vi "Read Array Of Tag Elements.vi"(6 "error text in":string, 8 "error in":errorcluster, 10 "tag name":string, 11 "node in":refnum<k20>) -> (0 "error out":errorcluster, 3 "array of elements":refnum<k20>[](array[refnum]))   [LabVIEW 2020, in "AIM ARINC 664 Import.lvlib"]
uses:
  AIM ARINC 664 Import.lvlib
  <resource>/objmgr/DOMUserDefRef.rc
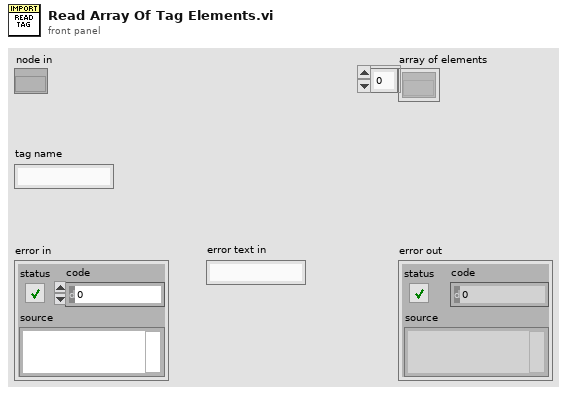
[diagram p1: front panel]
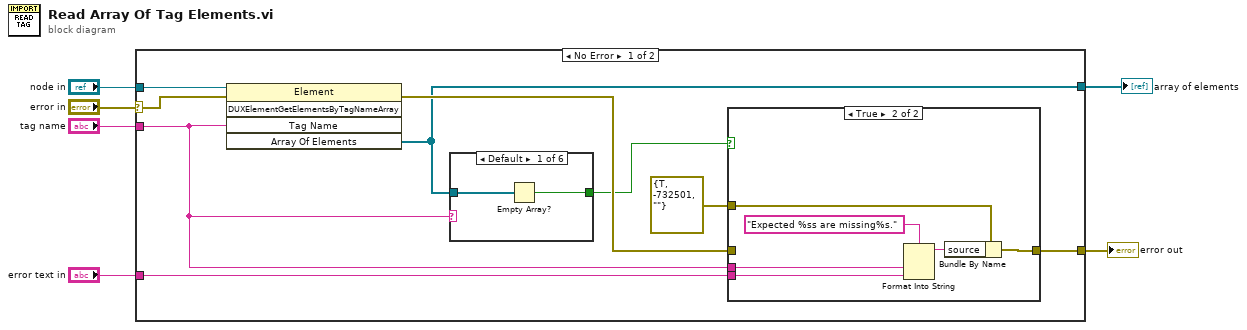
[diagram p0: block diagram]
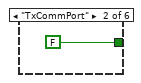
[diagram p2: hidden frame]
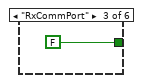
[diagram p3: hidden frame]
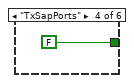
[diagram p4: hidden frame]
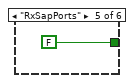
[diagram p5: hidden frame]
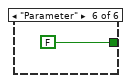
[diagram p6: hidden frame]
diagram:
  n1 = case shown="No Error" "error in" {
    selector: "error in" -> [w12 w30]
    tunnel: [w15 w30] -> w5
    tunnel: [w8 _] -> w4
    tunnel: "node in" -> [w13 _]
    tunnel: "tag name" -> [w9 _]
    tunnel: "error text in" -> [w10 _]
    frame No Error {
      n2 = invoke class="Element" method="DUXElementGetElementsByTagNameArray"(reference=w13, error in=w12, "Tag Name"=w9) -> (error out=w11:errorcluster, "Array Of Elements"=w8:refnum<k20>[])  [unwired: 2 in, 3 out]
      n3 = case shown="Default" w9 {
        tunnel: w8 -> [w17 _ _ _ _ _]
        tunnel: [w16 FALSE ("empty?") FALSE ("empty?") FALSE ("empty?") FALSE ("empty?") FALSE ("empty?")] -> w7
        frame Default {
          n4 = Empty Array?(array=w17) -> (empty?=w16:bool)
        }
        frame "TxCommPort" {
        }
        frame "RxCommPort" {
        }
        frame "TxSapPorts" {
        }
        frame "RxSapPorts" {
        }
        frame "Parameter" {
        }
      }
      n5 = case shown="True" w7 {
        tunnel: errorcluster {"status"=TRUE, "code"=-732501, "source"=""} ("error constant") -> [_ w28]
        tunnel: [w23 w29] -> w15
        tunnel: w11 -> [w23 _]
        tunnel: w9 -> [_ w26]
        tunnel: w10 -> [_ w24]
        frame False {
        }
        frame True {
          n6 = Format Into String(format string="Expected %ss are missing%s." ("source"), w26, w24) -> (resulting string=w27:string)  [unwired: 2 in, 1 out]
          n7 = Bundle By Name(cluster=w28, "source"=w27) -> (w29:errorcluster)
        }
      }
    }
    frame Error {
    }
  }
  "error out" <- w5
  "array of elements" <- w4
